vi "read_gr.vi"(4 "error in":errorcluster, 7 "datalog path":path) -> (0 "error out":errorcluster, 1 "DevNo":i32, 2 "group name":string, 3 "new file path":path)   [LabVIEW 2010]
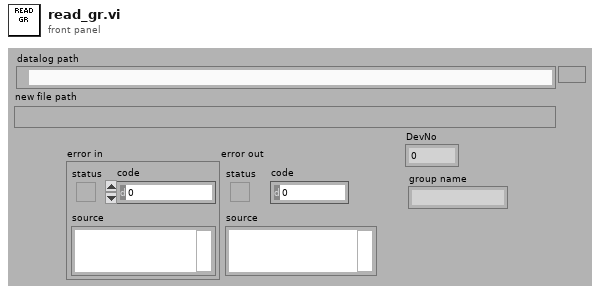
[diagram p1: front panel]
types:
  T1 = enum16{"open", "open or create", "create or replace", "create", "open (read-only)"}
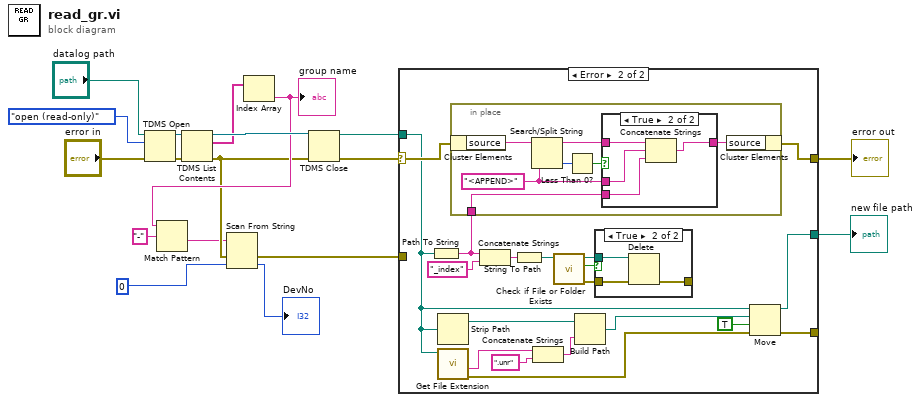
[diagram p0: block diagram]
diagram:
  n1 = TDMS Open(8:"error in", 10:T1."open (read-only)" ("operation (0:open)"), 11:"datalog path") -> (0:w15:errorcluster, 3:w16:refnum<k34>)  [unwired: 3 in]
  n2 = TDMS List Contents(4:w15, 7:w16) -> (0:w5:errorcluster, 2:w13:string[], 3:w14:refnum<k34>)  [unwired: 1 in, 1 out]
  n3 = Index Array(array=w13) -> (element=w8:string)  [unwired: 1 in]
  "group name" <- w8
  n4 = Match Pattern(string=w8, regular expression="-") -> (after substring=w4:string)  [unwired: 1 in, 3 out]
  n5 = Scan From String(input string=w4, error in=w5, default 1=0) -> (error out=w6:errorcluster, output 1=→"DevNo":i32)  [unwired: 2 in, 2 out]
  n6 = TDMS Close(8:w5, 11:w14) -> (0:w11:errorcluster, 3:w10:path)
  n7 = case shown="Error" w11 {
    selector: w11 -> [w20 w33]
    tunnel: [w20 w32] -> w1
    tunnel: [_ w24] -> _
    tunnel: w10 -> [w19 w22]
    tunnel: [w19 w21] -> w9
    tunnel: w6 -> [_ _]
    frame No Error {
    }
    frame Error {
      n8 = Path To String(path=w22) -> (string=w31:string)
      n9 = Strip Path(path=w22) -> (stripped path=w23:path)  [unwired: 1 out]
      n10 = call <vilib>:"Get File Extension.vi"("file"=w22) -> ("error out"=w26:errorcluster, "filename without extension"=w30:string)  [unwired: 7 in, 2 out]
      n11 = in-place {
        in-place-border: w31 -> [w41]
        w42 = "<APPEND>" ("regular expression")
        n12 = in-place-cluster #1(w33) -> ("source"=w46:string)
        n13 = Search/Split String(string=w46, search string/char (-)=w42) -> (substring before match=w43:string, offset of match=w45:i32)  [unwired: 1 in, 1 out]
        n14 = Less Than 0?(x=w45) -> (x < 0?=w44:bool)
        n15 = case shown="True" w44 {
          tunnel: w43 -> [w47 w51]
          tunnel: w42 -> [_ w50]
          tunnel: w41 -> [_ w49]
          tunnel: [w47 w48] -> w40
          frame False {
          }
          frame True {
            n16 = Concatenate Strings(w51, w50, w49) -> (w48:string)
          }
        }
        n17 = in-place-cluster #1("source"=w40) -> (w32:errorcluster)
      }
      n18 = Concatenate Strings(w31, "_index" ("string")) -> (w36:string)
      n19 = String To Path(string=w36) -> (path=w34:path)
      n20 = Concatenate Strings(w30, ".unr" ("string")) -> (w28:string)
      n21 = call <vilib>:"Check if File or Folder Exists.vi"("path"=w34) -> ("error out"=w38:errorcluster, "file or folder exists?"=w37:bool, "dup path"=w39:path)  [unwired: 8 in]
      n22 = Build Path(base path=w23, name or relative path=w28) -> (appended path=w27:path)
      n23 = case shown="True" w37 {
        tunnel: w39 -> [_ w54]
        tunnel: w38 -> [_ w53]
        tunnel: [_ w52] -> _
        frame False {
        }
        frame True {
          n24 = Delete(path (use dialog)=w54, error in=w53) -> (error out=w52:errorcluster)  [unwired: 3 in, 2 out]
        }
      }
      n25 = Move(source path=w22, error in=w26, 9:TRUE ("overwrite (F)"), 10:w27) -> (error out=w24:errorcluster, 3:w21:path)  [unwired: 1 in, 1 out]
    }
  }
  "error out" <- w1
  "new file path" <- w9
